vi "20T_Change_lambda_Control_Status.vi"(8 "error in (no error)":errorcluster, 10 "20 T Magnet control":T1={"Clamp"=FALSE, "Switch Heater"=FALSE, "Go to Zero"=FALSE, "Go to Set"=FALSE, "Go to Hold"=FALSE, "Field Setpoint (T)"=3.4572, "Rate Setpoint (T/min)"=0.0, "Set Rate"=FALSE, "Activate lambda control"=FALSE, "Set lambda NV"=FALSE, "lambda NV  SP"=3.4572} {"lambda NV  SP" format="%.1f"; "Rate Setpoint (T/min)" format="%6_5f"; "Field Setpoint (T)" format="%#4_5f"}, 11 "Mercury Reference In":T2) -> (0 "error out":errorcluster)   [LabVIEW 2019]
uses:
  Equipment/Mercury iXX/Public/Controls/Mercury Reference.ctl
  Equipment/Mercury iXX/Public/Controls/Comms Transport Layer.ctl
  Equipment/Mercury iXX/Private/Controls/Query Dynamic Reference.ctl
  Monitor Communication/Gustav/20T_Control.ctl
  Equipment/Mercury iXX/Public/Libraries/Lambda/Open/Open Lambda Device.vi
  Equipment/Mercury iXX/Mercury iXX.lvlib
  Equipment/Mercury iXX/Public/Libraries/Lambda.lvlib
panel:
  # "20 T"
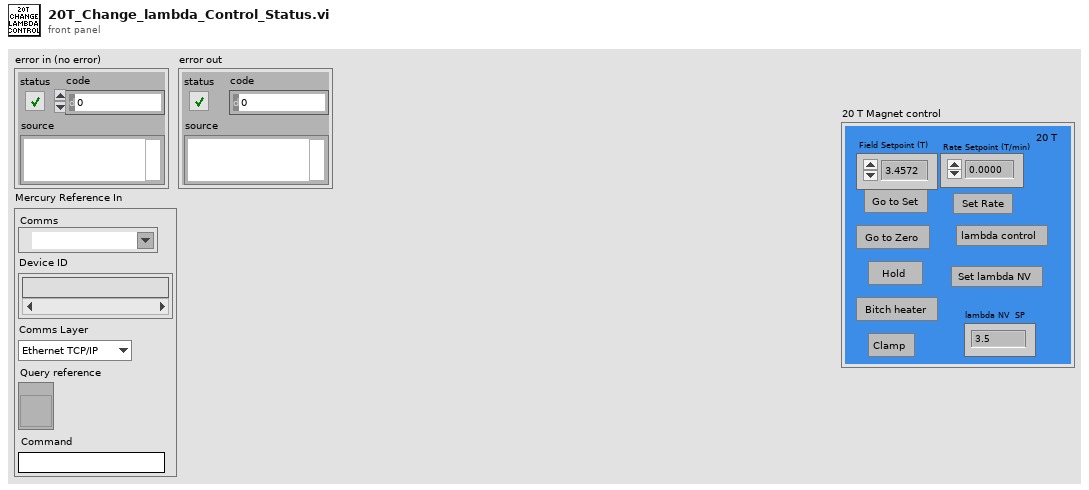
[diagram p1: front panel]
types:
  T1 = typedef "20T_Control.ctl" = cluster{"Clamp":bool, "Switch Heater":bool, "Go to Zero":bool, "Go to Set":bool, "Go to Hold":bool, "Field Setpoint (T)":dbl, "Rate Setpoint (T/min)":dbl, "Set Rate":bool, "Activate lambda control":bool, "Set lambda NV":bool, "lambda NV  SP":dbl}
  T2 = typedef "Mercury iXX.lvlib/Mercury Reference.ctl" = cluster{"Comms":refnum<visa-resource-name>, "Device ID":string[], "Comms Layer":T3, "Command":string, "Query reference":T4}
  T3 = typedef "Mercury iXX.lvlib/Comms Transport Layer.ctl" = enum16{"Ethernet TCP/IP", "USB", "ISOBus - RS-232", "GPIB"}
  T4 = typedef "Mercury iXX.lvlib/Query Dynamic Reference.ctl" = refnum<vi>
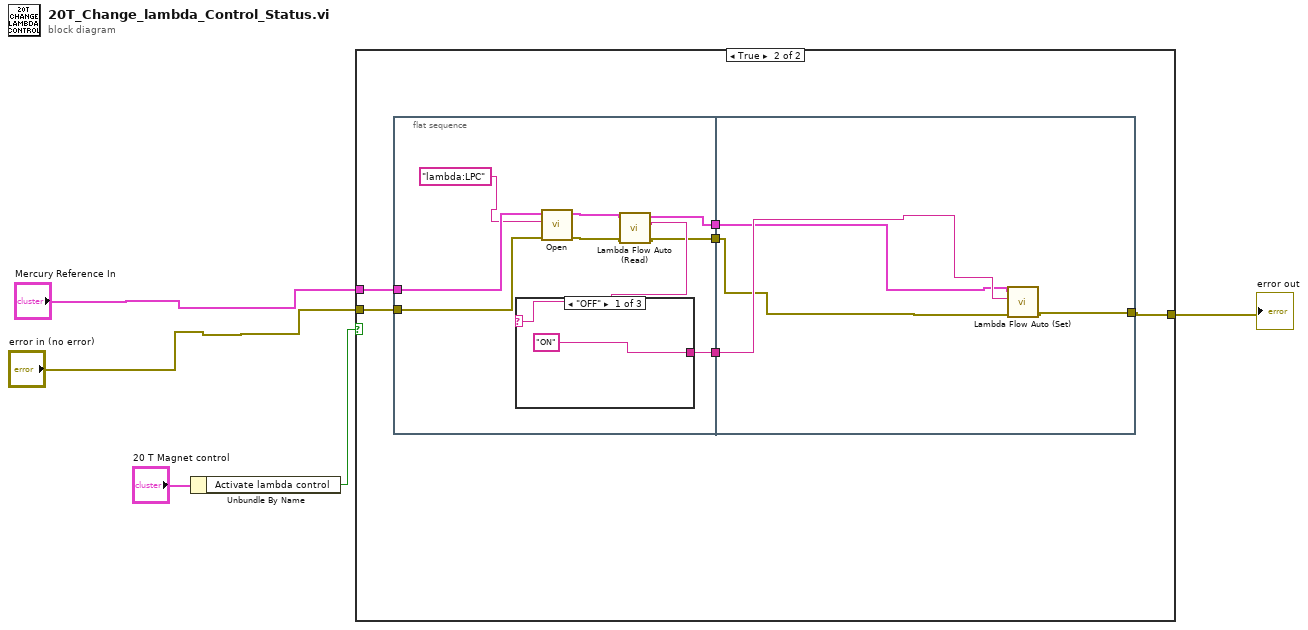
[diagram p0: block diagram]
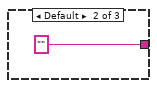
[diagram p3: hidden frame]
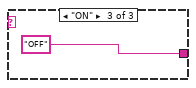
[diagram p4: hidden frame]
diagram:
  n1 = Unbundle By Name("20 T Magnet control") -> ("Activate lambda control"=w1:bool)
  n2 = case shown="True" w1 {
    tunnel: [w6 w10] -> w5
    tunnel: "Mercury Reference In" -> [_ w9]
    tunnel: "error in (no error)" -> [w6 w8]
    frame False {
    }
    frame True {
      n3 = flat-sequence {
        tunnel: w9 -> [w21]
        tunnel: w8 -> [w20]
        tunnel: [w14] -> w12
        tunnel: [w19] -> w11
        tunnel: [w13] -> w7
        tunnel: w12 -> [w25]
        tunnel: w11 -> [w28]
        tunnel: [w27] -> w10
        tunnel: w7 -> [w26]
        frame #0 {
          n4 = call-poly "Open.vi"("error in (no error)"=w20, "Device Identifier"="lambda:LPC", "Mercury Reference In"=w21) -> ("error out"=w16:errorcluster, "Mercury Reference Out"=w17:T2)  [unwired: 1 in, 6 out]
          n5 = call "Lambda Flow Auto (Read).vi"("error in"=w16, "Mercury Reference In"=w17) -> ("error out"=w14:errorcluster, "Lambda Auto"=w15:string, "Mercury Reference Out"=w13:T2)  [unwired: 6 in, 1 out]
          n6 = case shown="\"OFF\"" w15 {
            tunnel: ["ON" "" "OFF"] -> w19
            frame "OFF" {
            }
            frame Default {
            }
            frame "ON" {
            }
          }
        }
        frame #1 {
          n7 = call "Lambda Flow Auto (Set).vi"("error in"=w25, "Lambda Auto"=w28, "Mercury Reference In"=w26) -> ("error out"=w27:errorcluster)  [unwired: 5 in, 3 out]
        }
      }
    }
  }
  "error out" <- w5
